vi "USG_Query PROP.vi"(0 "System no.":i32=1 min=1 max=4 step=1, 5 "error in":errorcluster) -> (14 "List of System Properties":string, 19 "error out":errorcluster)   [LabVIEW 2020]
doc: "USG? PROP (System Properties) \n\nDescription\nOutputs the \"PROP\" section of the user guide.\nThe \"PROP\" section contains information on the properties of the existing container units and \nfunction units (p. 91). Depending on the argument(s) used, the display is limited to certain units.\n\nFormat\nUSG? PROP[ <Container Unit>[ <Function Unit>]]\n\nArguments\n<Container Unit>\nContainer unit\nPossible values: Alias of the container unit (p. 94) \n<Function Unit>\nFunction unitIf <Function Unit> is not specified, information about all function units contained \nin the container unit are output.\nIf only information about a certain container unit are to be displayed, \"-\" must be entered for \n<Function Unit>. \nPossible values:\nAlias of the function unit (p. 94) \n\"-\" \n\nResponse\nThe output always has the following format: \nThe Unit Properties block consists of at least the following fields:\n- Container Unit Alias (p. 94) for the container unit\n- Function Unit Alias (p. 94) for the function unit. The value \"-\" means that the \ndescription refers to the container unit.\n- Description Description of the container unit or function unit.\n- Additionally, at least one block with properties of the unit can be included, e.g. \n#Operation Modes (for axes), #Recordable Parameter Types (for data recorders) or \n#User Command Level (for interpreters).\n\nNotes\nUSG? without any arguments (p. 72) displays the contents of the user guide, i.e. the titles of the \navailable sections.\n\nUser command level\nUSR"
panel:
  # "USG? PROP (System Properties) \n\nOutputs the \"PROP\" section of the user guide.\nThe \"PROP\" section contains information on the properties of the existing container units and function units. Depending on the argument(s) used, the display is limited to certain units."
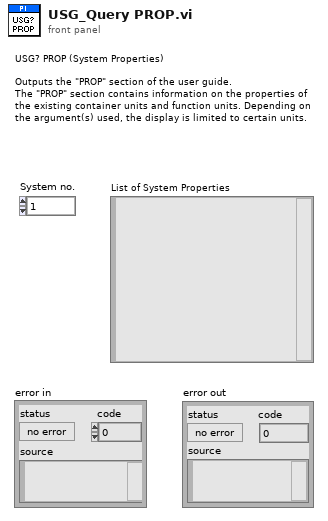
[diagram p1: front panel]
types:
  T1 = typedef "Syntax.ctl" = enum16{"GCS 1.0", "GCS 2.0", "GCS 3.0"}
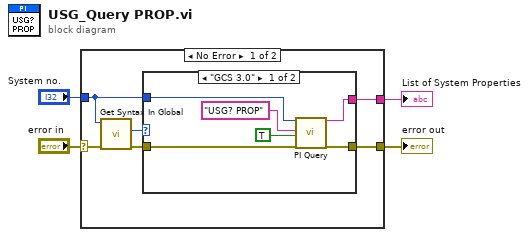
[diagram p0: block diagram]
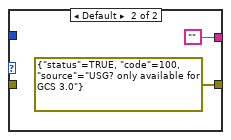
[diagram p2: hidden frame]
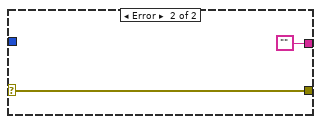
[diagram p3: hidden frame]
diagram:
  n1 = case shown="No Error" "error in" {
    selector: "error in" -> [w9 w20]
    tunnel: [w10 w20] -> w2
    tunnel: "System no." -> [w6 _]
    tunnel: [w5 ""] -> w1
    frame No Error {
      n2 = call "Get Syntax In Global.vi"("error in"=w9, "System no."=w6) -> ("error out"=w8:errorcluster, "Syntax"=w7:T1)  [unwired: 8 in]
      n3 = case shown="\"GCS 3.0\"" w7 {
        tunnel: [w11 errorcluster {"status"=TRUE, "code"=100, "source"="USG? only available for GCS 3.0"} ("error out")] -> w10
        tunnel: w6 -> [w16 _]
        tunnel: w8 -> [w15 _]
        tunnel: [w12 ""] -> w5
        frame "GCS 3.0" {
          n4 = call "PI Query.vi"("System no."=w16, "String to send"="USG? PROP", "Attach termination char.?"=TRUE, "error in"=w15) -> ("String read"=w12:string, "error out"=w11:errorcluster)  [unwired: 12 in, 2 out]
        }
        frame Default {
        }
      }
    }
    frame Error {
    }
  }
  "error out" <- w2
  "List of System Properties" <- w1
